vi "ACT_LabVIEW4_Task1B_Team072.vi"() -> ()   [LabVIEW 2016]
uses:
  <vilib>/express/express arith-compare/Formula/XNode/ExpressFormulaBlockNode.xnode
panel:
  out "t":dbl
  in  "r":dbl
  in  "m":dbl
  in  "h, height":dbl
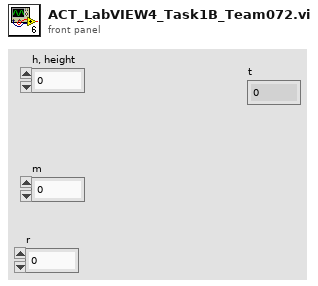
[diagram p1: front panel]
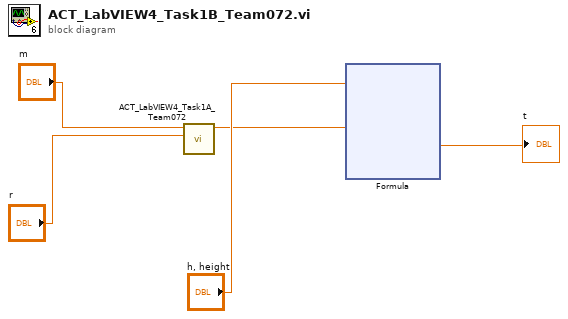
[diagram p0: block diagram]
diagram:
  n1 = call "ACT_LabVIEW4_Task1A_Team072.vi"("r, radius (m)"="r", "m, mass (kg)"="m") -> ("g, acceleration due to gravity"=w2:dbl)  [unwired: 9 in]
  n2 = xnode "Formula"("g"=w2, "h"="h, height") -> ("Result"=→"t":dbl)  [unwired: 1 in, 1 out]
